vi "Gripper Timer.vi"(2 "Target Time (s)":dbl, 3 "Reset Timer":bool) -> (0 "Elapsed Time":dbl, 1 "Time Reached?":bool)   [LabVIEW 2018]
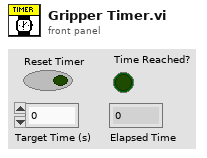
[diagram p1: front panel]
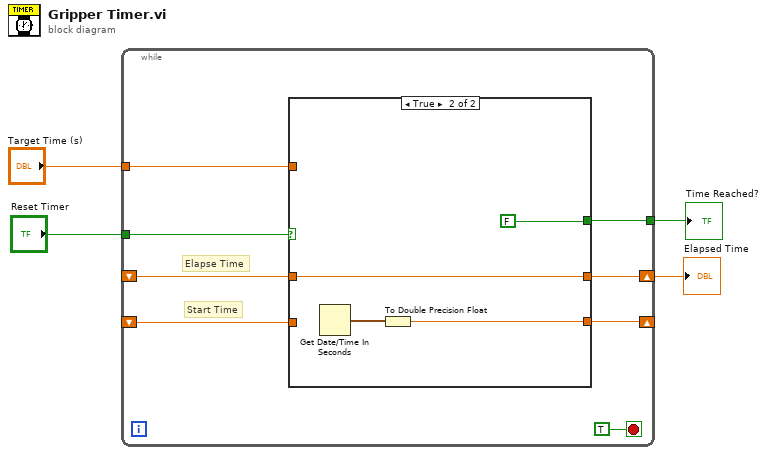
[diagram p0: block diagram]
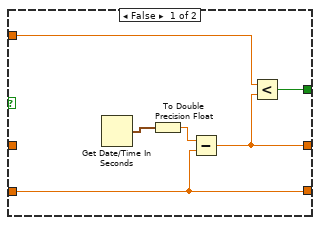
[diagram p2: hidden frame]
diagram:
  n1 = while {
    tunnel: "Reset Timer" -> [w11]
    shift-right: [w8] -> w1
    shift-left: _ -> [w5]
    shift-right: [w10] -> _
    shift-left: _ -> [w9]
    tunnel: [w7] -> w3
    tunnel: "Target Time (s)" -> [w6]
    stop <- TRUE stop-if-true
    # "Start Time"
    # "Elapse Time"
    n2 = case shown="True" w11 {
      tunnel: [w18 w21] -> w10
      tunnel: w9 -> [w18 _]
      tunnel: w5 -> [_ w20]
      tunnel: [w16 w20] -> w8
      tunnel: [w15 FALSE] -> w7
      tunnel: w6 -> [w14 _]
      frame False {
        n3 = Get Date/Time In Seconds() -> (seconds since 1Jan1904=w13:timestamp)
        n4 = To Double Precision Float(number=w13) -> (double precision float=w17:dbl)
        n5 = Subtract(x=w17, y=w18) -> (x-y=w16:dbl)
        n6 = Less?(x=w14, y=w16) -> (x < y?=w15:bool)
      }
      frame True {
        n7 = Get Date/Time In Seconds() -> (seconds since 1Jan1904=w22:timestamp)
        n8 = To Double Precision Float(number=w22) -> (double precision float=w21:dbl)
      }
    }
  }
  "Elapsed Time" <- w1
  "Time Reached?" <- w3
